vi "Panel Resize.vi"(8 "error in (no error)":errorcluster, 11 "CheckPasswordUI in":refnum<class "CheckPasswordUI.lvclass">) -> (0 "error out":errorcluster, 3 "CheckPasswordUI out":refnum<class "CheckPasswordUI.lvclass">)   [LabVIEW 2021, in "CheckPasswordUI.lvclass"]
uses:
  CheckPasswordUI.lvclass
  C:/Program Files (x86)/National Instruments/LabVIEW 2021/user.lib/John_Lib/AbstractActorTemplate/AbstractActorTemplate/UIActorTop.lvclass
  CheckPasswordUI.lvclass/CheckPasswordUI.ctl
panel:
  in  "s":bool
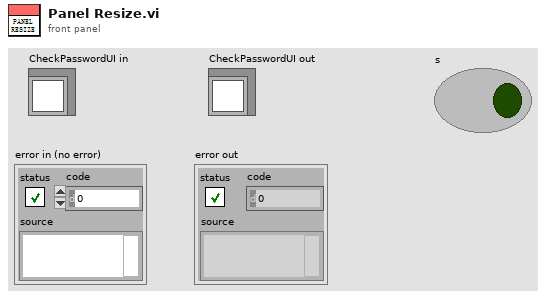
[diagram p1: front panel]
types:
  T1 = typedef "LVRectTypeDef.ctl" = cluster{"Left":i16, "Top":i16, "Right":i16, "Bottom":i16}
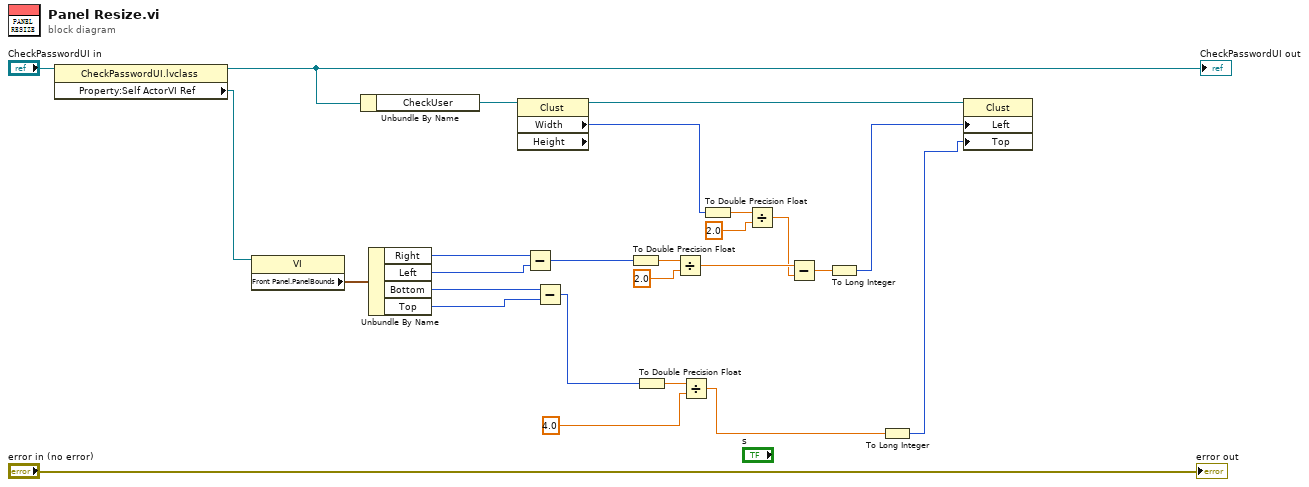
[diagram p0: block diagram]
diagram:
  n1 = property class="CheckPasswordUI.lvclass"(reference="CheckPasswordUI in") -> (reference out=w18:refnum<class "CheckPasswordUI.lvclass">, "Property:Self ActorVI Ref"=w24:refnum<vi>)  [unwired: 1 in, 1 out]
  "CheckPasswordUI out" <- w18
  n2 = property class="VI"(reference=w24) -> ("Front Panel.PanelBounds"=w23:T1)  [unwired: 1 in, 2 out]
  n3 = Unbundle By Name(w18) -> ("CheckUser"=w14:refnum<vi>)
  n4 = Unbundle By Name(w23) -> ("Right"=w22:i16, "Left"=w21:i16, "Bottom"=w20:i16, "Top"=w19:i16)
  n5 = property class="Clust" props=["Width", "Height"](reference=w14) -> (reference out=w13:refnum<vi>, "Width"=w10:u32)  [unwired: 1 in, 2 out]
  n6 = Subtract(x=w22, y=w21) -> (x-y=w17:i16)
  n7 = Subtract(x=w20, y=w19) -> (x-y=w3:i16)
  n8 = To Double Precision Float(number=w17) -> (double precision float=w16:dbl)
  n9 = To Double Precision Float(number=w3) -> (double precision float=w4:dbl)
  n10 = Divide(x=w16, y=2.0) -> (x/y=w9:dbl)
  n11 = Divide(x=w4, y=4.0) -> (x/y=w1:dbl)
  n12 = To Double Precision Float(number=w10) -> (double precision float=w11:dbl)
  n13 = Divide(x=w11, y=2.0) -> (x/y=w8:dbl)
  n14 = Subtract(x=w9, y=w8) -> (x-y=w7:dbl)
  n15 = To Long Integer(number=w7) -> (32bit integer=w6:i32)
  n16 = To Long Integer(number=w1) -> (32bit integer=w2:i32)
  n17 = property class="Clust"(reference=w13, "Left"=w6, "Top"=w2) -> ()  [unwired: 1 in, 2 out]
  "error out" <- "error in (no error)"
